vi "Initialize-status-notifiers.vi"(8 "error in (no error)":errorcluster, 11 "ModComm in":T1) -> (0 "error out":errorcluster, 3 "ModComm out":T1)   [LabVIEW 2013, in "Server.lvlib" / "Server.lvclass"]
uses:
  Server.lvclass
  Object-reference.ctl
  Server.lvclass/Server.ctl
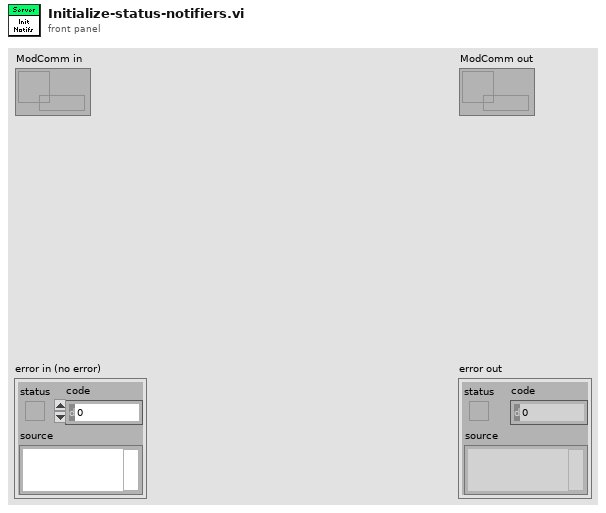
[diagram p1: front panel]
types:
  T1 = typedef "Server.lvlib/Server.lvclass/Object-reference.ctl" = refnum<data-value>
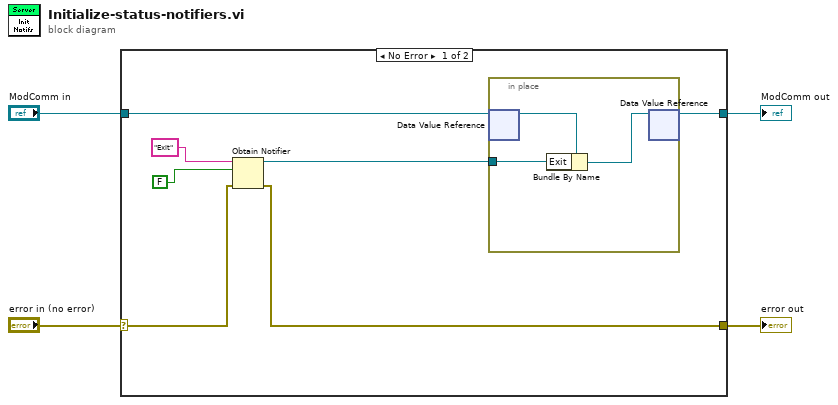
[diagram p0: block diagram]
diagram:
  n1 = case shown="No Error" "error in (no error)" {
    selector: "error in (no error)" -> [w9 w16]
    tunnel: [w8 w16] -> w3
    tunnel: [w5 w15] -> w1
    tunnel: "ModComm in" -> [w7 w15]
    frame No Error {
      n2 = Obtain Notifier(name (unnamed)="Exit", notification data type=FALSE, error in (no error)=w9) -> (notifier out=w6:refnum<notifier>, error out=w8:errorcluster)  [unwired: 1 in, 1 out]
      n3 = in-place {
        in-place-border: w6 -> [w14]
        n4 = in-place-dvr #1(w7) -> (w13:refnum<class "Server.lvclass">)  [unwired: 1 out]
        n5 = Bundle By Name(cluster=w13, "Exit"=w14) -> (w12:refnum<class "Server.lvclass">)
        n6 = in-place-dvr #1(w12) -> (w5:T1)  [unwired: 1 out]
      }
    }
    frame Error {
    }
  }
  "error out" <- w3
  "ModComm out" <- w1
